vi "D-Lockin.vi"(8 "error in (no error)":errorcluster, 9 "index":u32, 10 "Stop?":bool, 11 "SweepControl":refnum<class "SweepControl.lvclass">) -> (0 "error out":errorcluster, 3 "SweepControl":refnum<class "SweepControl.lvclass">)   [LabVIEW 2016, in "SweepControl.lvclass"]
uses:
  SweepControl/SweepControl.lvclass
  SweepControl/SweepControl.lvclass/SweepControl.ctl
  Transport.lvclass
  <userlib>/LevyLab/LV to ITX/LVtoITX.lvclass
panel:
  in  "V2":i32=1 min=1
  in  "V1":i32=1 min=1
  in  "Current":i32=1 min=1
  out "G4T":cluster{dbl[], dbl[]}[](graph)
  out "Y Lockins":cluster{dbl[], dbl[]}[](graph)
  out "X Lockins":cluster{dbl[], dbl[]}[](graph)
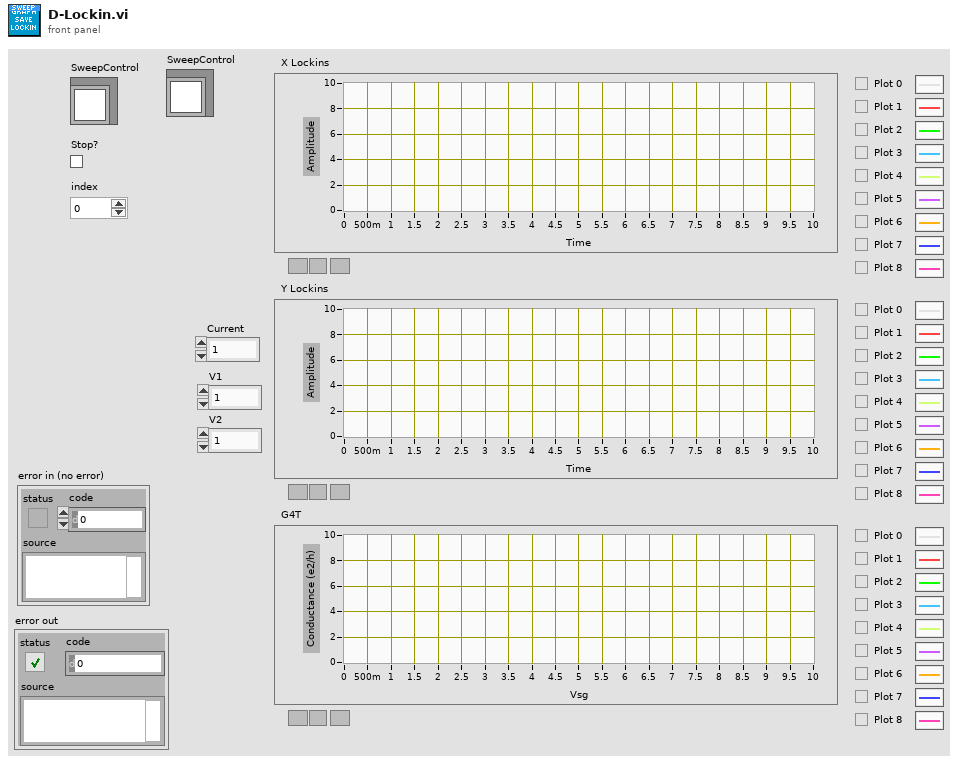
[diagram p1: front panel]
types:
  T1 = cluster{"path":path, "Experiment Folder":string, "device":string, "Comments":string}
  T2 = cluster{"Result X":dbl[], "Result Y":dbl[], "Data":cluster{"Y  Array":dbl[]}[], "wavenames":string[], "All Result X":dbl[][], "All Result Y":dbl[][]}
  T3 = cluster{"SweepControl":refnum<class "SweepControl.lvclass">, "file":cluster{"path":path, "Experiment Folder":string, "device":string, "Comments":string}, "data":cluster{"Result X":dbl[], "Result Y":dbl[], "Data":cluster{"Y  Array":dbl[]}[], "wavenames":string[], "All Result X":dbl[][], "All Result Y":dbl[][]}, "lockin address":string, "All Parameters":dbl[]}
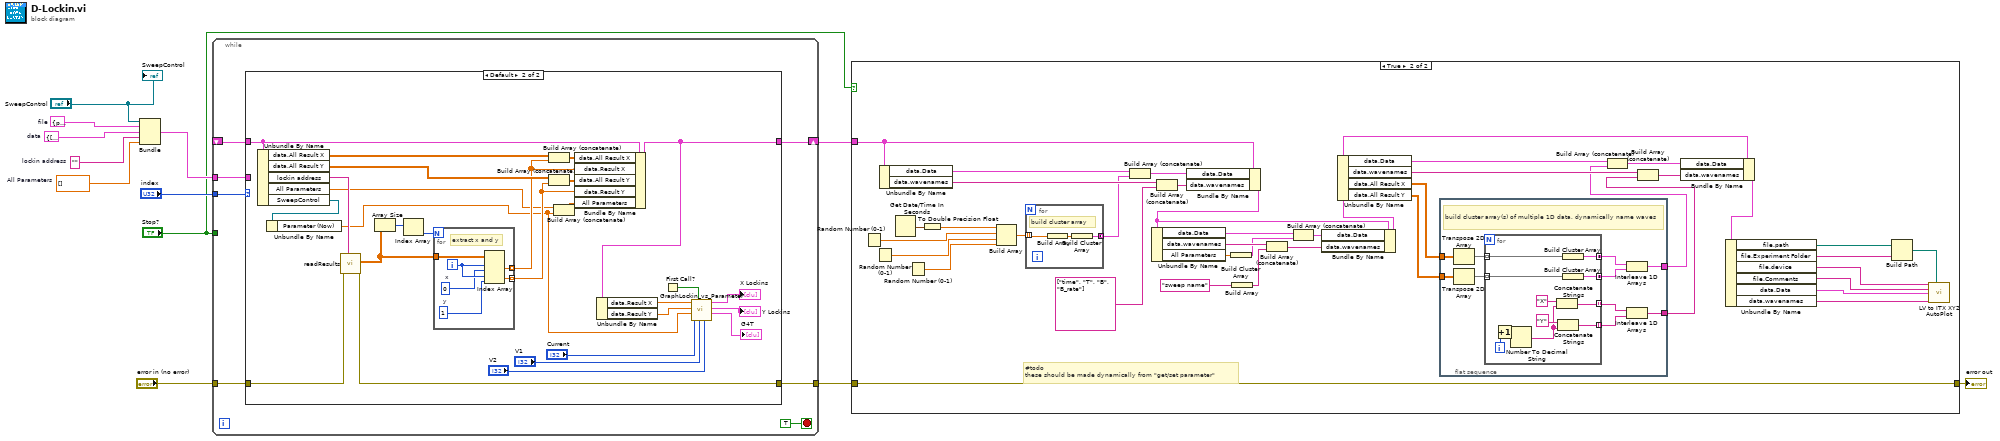
[diagram p0: block diagram]
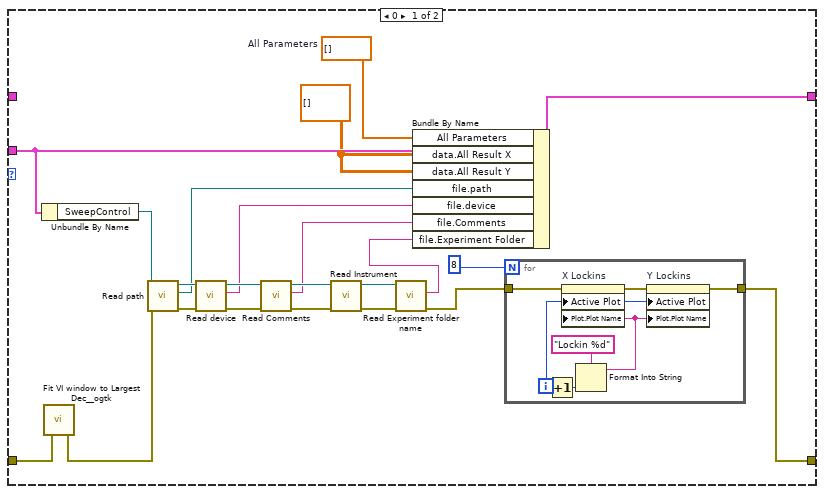
[diagram p3: hidden frame]
diagram:
  w3 = dbl[] []  # All Parameters
  w6 = ""  # lockin address
  w8 = T1 {"path"=path "", "Experiment Folder"="", "device"="", "Comments"=""}  # file
  w7 = T2 {"Result X"=[], "Result Y"=[], "Data"=[], "wavenames"=[], "All Result X"=[], "All Result Y"=[]}  # data
  n1 = Bundle("SweepControl"="SweepControl", "file"=w8, "data"=w7, "lockin address"=w6, "All Parameters"=w3) -> (w9:T3)  [unwired: 1 in]
  n2 = while {
    tunnel: "index" -> [w19]
    tunnel: "Stop?" -> [_]
    tunnel: "error in (no error)" -> [w18]
    shift-right: [w16] -> w4
    shift-left: _ -> [w17]
    tunnel: w9 -> [w15]
    tunnel: [w14] -> w2
    stop <- TRUE stop-if-true
    n3 = case shown="Default" w19 {
      tunnel: w18 -> [w25 w65]
      tunnel: w17 -> [_ w63]
      tunnel: [w31 w61] -> w16
      tunnel: w15 -> [w30 _]
      tunnel: [w26 w64] -> w14
      frame 0 {
        w21 = dbl[] []  # All Parameters
        w22 = dbl[][] [] ("data.All Result X")
        n4 = Unbundle By Name(w30) -> ("SweepControl"=w32:refnum<class "SweepControl.lvclass">)
        n5 = call <userlib>:"Fit VI window to Largest Dec__ogtk.vi"("error in (no error)"=w25) -> ("error out"=w24:errorcluster)  [unwired: 5 in, 1 out]
        n6 = call-dynamic "Read path.vi"("error in (no error)"=w24, "SweepControl in"=w32) -> ("error out"=w40:errorcluster, "path"=w35:path, "SweepControl out"=w41:refnum<class "SweepControl.lvclass">)  [unwired: 7 in]
        n7 = call-dynamic "Read device.vi"("error in (no error)"=w40, "SweepControl in"=w41) -> ("error out"=w39:errorcluster, "device"=w34:string, "SweepControl out"=w38:refnum<class "SweepControl.lvclass">)  [unwired: 7 in]
        n8 = call-dynamic "Read Comments.vi"("error in (no error)"=w39, "SweepControl in"=w38) -> ("error out"=w36:errorcluster, "Comments"=w33:string, "SweepControl out"=w37:refnum<class "SweepControl.lvclass">)  [unwired: 7 in]
        n9 = call-dynamic "Read Instrument.vi"("error in (no error)"=w36, "SweepControl in"=w37) -> ("error out"=w29:errorcluster, "SweepControl out"=w28:refnum<class "SweepControl.lvclass">)  [unwired: 7 in, 1 out]
        n10 = call-dynamic "Read Experiment folder name.vi"("error in (no error)"=w29, "SweepControl in"=w28) -> ("error out"=w23:errorcluster, "Experiment folder name"=w20:string)  [unwired: 7 in, 1 out]
        n11 = Bundle By Name(cluster=w30, "All Parameters"=w21, "data.All Result X"=w22, "data.All Result Y"=w22, "file.path"=w35, "file.device"=w34, "file.Comments"=w33, "file.Experiment Folder"=w20) -> (w31:T3)
        n12 = for {
          N: 8 -> [_]
          tunnel: [w43] -> w26
          tunnel: w23 -> [w42]
          i -> [w46]
          n13 = Increment(x=w46) -> (x+1=w44:i32)
          n14 = Format Into String(format string="Lockin %d", w44) -> (resulting string=w47:string)  [unwired: 2 in, 1 out]
          n15 = property on="X Lockins" class="XYGraph (strict)"(error in=w42, "Active Plot"=w46, "Plot.Plot Name"=w47) -> (error out=w45:errorcluster)  [unwired: 1 in, 1 out]
          n16 = property on="Y Lockins" class="XYGraph (strict)"(error in=w45, "Active Plot"=w46, "Plot.Plot Name"=w47) -> (error out=w43:errorcluster)  [unwired: 1 in, 1 out]
        }
      }
      frame Default {
        n17 = Unbundle By Name(w63) -> ("data.All Result X"=w72:dbl[][], "data.All Result Y"=w71:dbl[][], "lockin address"=w75:string, "All Parameters"=w55:dbl[], "SweepControl"=w54:refnum<class "SweepControl.lvclass">)
        n18 = Unbundle By Name(w54) -> ("Parameter (Now)"=w53:dbl)
        n19 = call <userlib>:"readResults.vi"("address"=w75, "error in (no error)"=w65) -> ("error out"=w64:errorcluster, "Results"=w66:dbl[][])  [unwired: 7 in, 1 out]
        n20 = Array Size(array=w66) -> (size(s)=w74:i32[])
        n21 = Index Array(array=w74) -> (element=w73:i32)  [unwired: 1 in]
        n22 = for {
          N: w73 -> [_]
          tunnel: w66 -> [w81]
          tunnel: [w79] -> w70 mode=indexing
          tunnel: [w78] -> w69 mode=indexing
          i -> [w80]
          w76 = 1  # y
          w77 = 0  # x
          # "extract x and y"
          n23 = Index Array(array=w81, index (row) #1=w80, index (col) #1=w77, index (row) #2=w80, index (col) #2=w76) -> (element #1=w79:dbl, element #2=w78:dbl)
        }
        n24 = Build Array (concatenate)(w72, w70) -> (w67:dbl[][])
        n25 = Build Array (concatenate)(w71, w69) -> (w68:dbl[][])
        n26 = Build Array (concatenate)(w55, w53) -> (w52:dbl[])
        n27 = Bundle By Name(cluster=w63, "data.All Result X"=w67, "data.Result X"=w70, "data.All Result Y"=w68, "data.Result Y"=w69, "All Parameters"=w52) -> (w61:T3)
        n28 = Unbundle By Name(w61) -> ("data.Result X"=w62:dbl[], "data.Result Y"=w59:dbl[])
        n29 = First Call?() -> (First Call?: T/F=w60:bool)
        n30 = call "GraphLockin_vs_Parameter.vi"("V2"="V2", "V1"="V1", "reset?"=w60, "Current"="Current", "Parameter"=w53, "Y[ ]"=w59, "X[ ]"=w62) -> ("G(e2/h) vs Parameter"=→"G4T":cluster{"Y":dbl[], "Y":dbl[]}[], "Y vs Parameter"=→"Y Lockins":cluster{dbl[], dbl[]}[], "X vs Parameter"=→"X Lockins":cluster{dbl[], dbl[]}[])  [unwired: 1 in, 1 out]
      }
    }
  }
  n31 = case shown="True" "Stop?" {
    tunnel: w4 -> [_ w113]
    tunnel: w2 -> [w82 w83]
    tunnel: [w82 w83] -> w1
    frame False {
    }
    frame True {
      # "#todo\nthese should be made dynamically from \"get/set parameter\""
      n32 = Random Number (0-1)() -> (number: 0 to 1=w112:dbl)
      n33 = Random Number (0-1)() -> (number: 0 to 1=w111:dbl)
      n34 = Unbundle By Name(w113) -> ("data.Data"=w122:cluster{"Y  Array":dbl[]}[], "data.wavenames"=w121:string[])
      n35 = Get Date/Time In Seconds() -> (seconds since 1Jan1904=w117:timestamp)
      n36 = Random Number (0-1)() -> (number: 0 to 1=w110:dbl)
      n37 = To Double Precision Float(number=w117) -> (double precision float=w116:dbl)
      n38 = Build Array(w116, w112, w111, w110) -> (w114:dbl[])
      n39 = for {
        tunnel: [w145] -> w115 mode=concatenating
        tunnel: w114 -> [w144] mode=indexing
        # "build cluster array"
        n40 = Build Array(w144) -> (w146:dbl[])
        n41 = Build Cluster Array(w146) -> (w145:cluster{dbl[]}[])
      }
      n42 = Build Array (concatenate)(w122, w115) -> (w119:cluster{"Y  Array":dbl[]}[])
      n43 = Build Array (concatenate)(w121, string[] ["time", "T", "B", "B_rate"] ("wavenames (.Vx, etc)")) -> (w120:string[])
      n44 = Bundle By Name(cluster=w113, "data.Data"=w119, "data.wavenames"=w120) -> (w93:T3)
      n45 = Unbundle By Name(w93) -> ("data.Data"=w109:cluster{"Y  Array":dbl[]}[], "data.wavenames"=w108:string[], "All Parameters"=w106:dbl[])
      n46 = Build Cluster Array(w106) -> (w105:cluster{"All Parameters":dbl[]}[])
      n47 = Build Array("sweep name" ("wavenames")) -> (w102:string[])
      n48 = Build Array (concatenate)(w108, w102) -> (w104:string[])
      n49 = Build Array (concatenate)(w109, w105) -> (w107:cluster{"All Parameters":dbl[]}[])
      n50 = Bundle By Name(cluster=w93, "data.Data"=w107, "data.wavenames"=w104) -> (w84:T3)
      n51 = Unbundle By Name(w84) -> ("data.Data"=w101:cluster{"Y  Array":dbl[]}[], "data.wavenames"=w100:string[], "data.All Result X"=w97:dbl[][], "data.All Result Y"=w96:dbl[][])
      n52 = flat-sequence {
        tunnel: w97 -> [w132]
        tunnel: w96 -> [w131]
        tunnel: [w124] -> w94
        tunnel: [w123] -> w95
        frame #0 {
          # "build cluster array(s) of multiple 1D data, dynamically name waves"
          n53 = Transpose 2D Array(2D array=w132) -> (transposed array=w130:dbl[][])
          n54 = Transpose 2D Array(2D array=w131) -> (transposed array=w129:dbl[][])
          n55 = for {
            tunnel: w130 -> [w143] mode=indexing
            tunnel: w129 -> [w142] mode=indexing
            tunnel: [w141] -> w128 mode=concatenating
            tunnel: [w140] -> w127 mode=concatenating
            tunnel: [w135] -> w126 mode=indexing
            tunnel: [w134] -> w125 mode=indexing
            i -> [w137]
            n56 = Increment(x=w137) -> (x+1=w133:i32)
            n57 = Number To Decimal String(number=w133) -> (decimal integer string=w136:string)  [unwired: 1 in]
            n58 = Concatenate Strings("X" ("wavenames"), w136) -> (w135:string)
            n59 = Concatenate Strings("Y" ("wavenames"), w136) -> (w134:string)
            n60 = Build Cluster Array(w143) -> (w141:cluster{dbl[]}[])
            n61 = Build Cluster Array(w142) -> (w140:cluster{dbl[]}[])
          }
          n62 = Interleave 1D Arrays(w128, w127) -> (w123:cluster{dbl[]}[])
          n63 = Interleave 1D Arrays(w126, w125) -> (w124:string[])
        }
      }
      n64 = Build Array (concatenate)(w101, w95) -> (w98:cluster{"Y  Array":dbl[]}[])
      n65 = Build Array (concatenate)(w100, w94) -> (w99:string[])
      n66 = Bundle By Name(cluster=w84, "data.Data"=w98, "data.wavenames"=w99) -> (w85:T3)
      n67 = Unbundle By Name(w85) -> ("file.path"=w86:path, "file.Experiment Folder"=w92:string, "file.device"=w90:string, "file.Comments"=w89:string, "data.Data"=w88:cluster{"Y  Array":dbl[]}[], "data.wavenames"=w87:string[])
      n68 = Build Path(base path=w86, name or relative path=w92) -> (appended path=w91:path)
      n69 = call <userlib>:"LV to ITX XY2 AutoPlot.vi"("filename"=w90, "path"=w91, "Notes"=w89, "Data"=w88, "wavenames (.Vx, etc)"=w87) -> ()  [unwired: 10 in, 1 out]
    }
  }
  "error out" <- w1
  "SweepControl" <- "SweepControl"
